vi "FT_Write.vi"(8 "error in (no error)":errorcluster, 10 "lpBuffer":u8[](array[numeric]) format="%.0x", 11 "ftHandle_in":u32 format="%.0x") -> (0 "error out":errorcluster, 1 "lpBytesWritten":u32, 2 "status":u32, 3 "ftHandle_out":u32 format="%.0x")   [LabVIEW 2019]
uses:
  FT_Error_codes.vi
  ftd2xx.dll
panel:
  out "lpBuffer_out":u8[](array[numeric]) format="%.0x"
  out "nBufferSize":u32
  in  "lpBytesWritten_in":i32
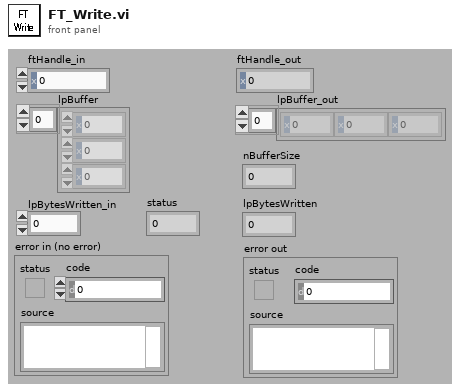
[diagram p1: front panel]
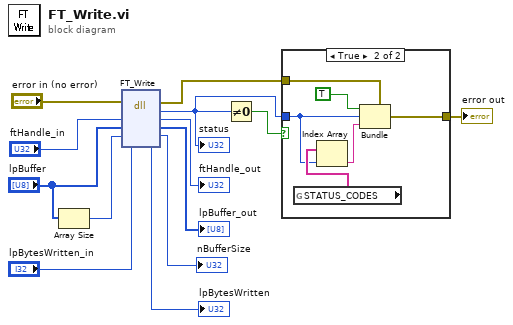
[diagram p0: block diagram]
diagram:
  n1 = Array Size(array="lpBuffer") -> (size(s)=w1:i32)
  n2 = dll-call lib="ftd2xx.dll" fn="FT_Write"(error in="error in (no error)", "ftHandle"="ftHandle_in", "lpBuffer"="lpBuffer", "nBufferSize"=w1, "lpBytesWritten"="lpBytesWritten_in") -> (error out=w10:errorcluster, "status"=w7:u32, "ftHandle"=→"ftHandle_out":u32, "lpBuffer"=→"lpBuffer_out":u8[], "nBufferSize"=→"nBufferSize":u32, "lpBytesWritten"=→"lpBytesWritten":u32)  [unwired: 2 in, 1 out]
  "status" <- w7
  n3 = Not Equal To 0?(x=w7) -> (x != 0?=w8:bool)
  n4 = case shown="True" w8 {
    tunnel: w10 -> [w14 w20]
    tunnel: [w14 w19] -> w9
    tunnel: w7 -> [_ w15]
    frame False {
    }
    frame True {
      n5 = global read "FT_Error_codes.vi" "STATUS_CODES"() -> (w16:string[])
      n6 = Index Array(array=w16, index=w15) -> (element=w17:string)
      n7 = Bundle(cluster=w20, "status"=TRUE, "code"=w15, "source"=w17) -> (w19:errorcluster)
    }
  }
  "error out" <- w9
